vi "coerce_to_ramp.vi"(0 "Requested speed\nvelocity units (% or native)":dbl format="%#_13g", 2 "Max Positive Acceleration\nvelocity units (% or native)/second":dbl=50.0 format="%#_13g", 3 "Max Positive Deceleration\nvelocity units (% or native)/second":dbl=50.0 format="%#_13g", 4 "Max Negative Acceleration\nvelocity units (% or native)/second":dbl=50.0 format="%#_13g", 5 "Max Negative Deceleration\nvelocity units (% or native)/second":dbl=50.0 format="%#_13g") -> (1 "Ramped speed\nvelocity units (% or native)/second":dbl format="%#_13g")   [LabVIEW 2017]
panel:
  in  "Teleop Loop Rate\n(seconds)":dbl=0.02 format="%#_13g"
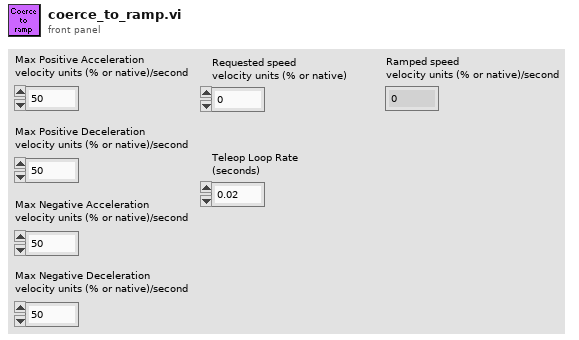
[diagram p1: front panel]
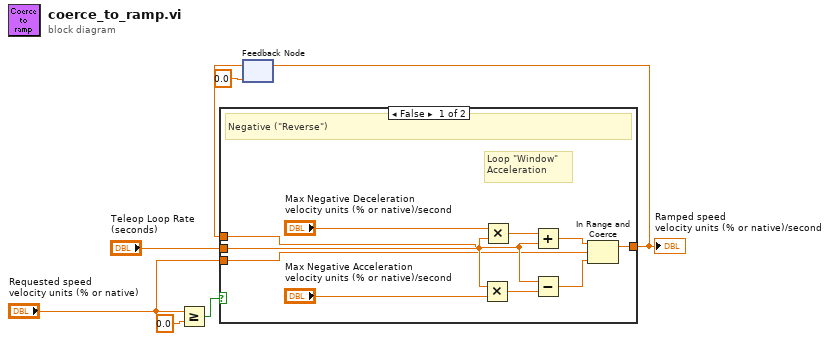
[diagram p0: block diagram]
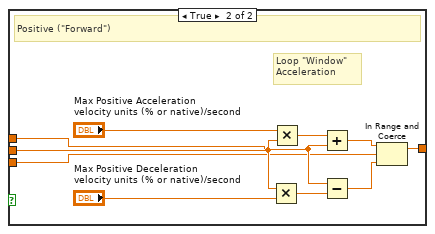
[diagram p2: hidden frame]
diagram:
  n1 = Greater Or Equal?(x="Requested speed\nvelocity units (% or native)", y=0.0) -> (x >= y?=w7:bool)
  n2 = feedback #1(0.0) -> (w5:dbl)
  n3 = case shown="False" w7 {
    tunnel: "Teleop Loop Rate\n(seconds)" -> [w11 w26]
    tunnel: [w14 w22] -> w3
    tunnel: w5 -> [w9 w21]
    tunnel: "Requested speed\nvelocity units (% or native)" -> [w8 w18]
    frame False {
      # "Loop \"Window\"\nAcceleration"
      # "Negative (\"Reverse\")"
      n4 = Multiply(x=w11, y="Max Negative Acceleration\nvelocity units (% or native)/second") -> (x*y=w15:dbl)
      n5 = Multiply(x="Max Negative Deceleration\nvelocity units (% or native)/second", y=w11) -> (x*y=w10:dbl)
      n6 = Add(x=w10, y=w9) -> (x+y=w17:dbl)
      n7 = Subtract(x=w9, y=w15) -> (x-y=w16:dbl)
      n8 = In Range and Coerce(upper limit=w17, x=w8, lower limit=w16) -> (coerced(x)=w14:dbl)  [unwired: 1 out]
    }
    frame True {
      # "Loop \"Window\"\nAcceleration"
      # "Positive (\"Forward\")"
      n9 = Multiply(x=w26, y="Max Positive Deceleration\nvelocity units (% or native)/second") -> (x*y=w19:dbl)
      n10 = Multiply(x="Max Positive Acceleration\nvelocity units (% or native)/second", y=w26) -> (x*y=w20:dbl)
      n11 = Add(x=w20, y=w21) -> (x+y=w23:dbl)
      n12 = Subtract(x=w21, y=w19) -> (x-y=w24:dbl)
      n13 = In Range and Coerce(upper limit=w23, x=w18, lower limit=w24) -> (coerced(x)=w22:dbl)  [unwired: 1 out]
    }
  }
  "Ramped speed\nvelocity units (% or native)/second" <- w3
  n14 = feedback-in #1(w3) -> ()
